vi "Session Request - Brose Session_2PORTS.vi"(0 "ID Request":string="18DA55F2", 1 "ID Response":string="18DAF255") -> (2 "Data String":string, 3 "ID String":string, 4 "Write":refnum<k21>, 5 "Read":refnum<k21>)   [LabVIEW 2023]
panel:
  out "error out":errorcluster
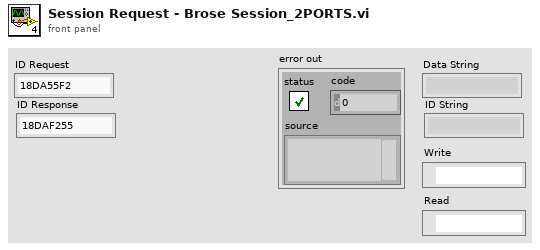
[diagram p1: front panel]
types:
  T1 = typedef "XNET Frame CAN.ctl" = cluster{"timestamp":timestamp, "payload":u8[], "identifier":u32, "type":T2, "extended?":bool, "echo?":bool}
  T2 = typedef "XNET Frame Type CAN.ctl" = u8
  T3 = cluster{"data[0]":T1, "data[1]":T1, "data[2]":T1, "data[3]":T1, "data[4]":T1, "data[5]":T1, "data[6]":T1, "data[7]":T1, "data[8]":T1}
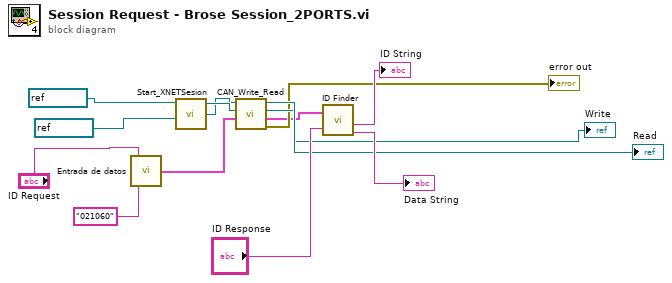
[diagram p0: block diagram]
diagram:
  n1 = call "Entrada de datos.vi"("string"="021060", "ID"="ID Request") -> ("CAN frame"=w7:T1)
  n2 = call "Start_XNETSesion.vi"("Read Interface"=refnum<k21> "CAN2", "Write Interface"=refnum<k21> "CAN1" ("interface")) -> ("Read"=w5:refnum<k21>, "Write"=w6:refnum<k21>)  [unwired: 2 in, 1 out]
  n3 = call "CAN_Write_Read.vi"("Read In"=w5, "Write In"=w6, "CAN frame"=w7) -> ("Read Out"=→"Read":refnum<k21>, "Write Out"=→"Write":refnum<k21>, "cluster"=w1:T3, "Error Out"=→"error out":errorcluster)  [unwired: 1 in, 1 out]
  n4 = call "ID Finder.vi"("cluster"=w1, "ID ESPERADO STRING"="ID Response") -> ("ID String"=→"ID String":string, "Data String"=→"Data String":string)  [unwired: 4 out]
